vi "ros data.vi"() -> ()   [LabVIEW 2015]
uses:
  Zmienne/szablon odometry_filtered_local.ctl
  TASK ERL/List of robots.ctl
  Zmienne/common msg from UAV-1.vi
  Gobal for ROS.vi
  Zmienne/Lokalizacja GPS/Longitude dron 2.vi
  Zmienne/Lokalizacja GPS/Latitude dron 2.vi
  Zmienne/Lokalizacja GPS/Longitude dron 1.vi
  Zmienne/Lokalizacja GPS/Latitude dron 1.vi
  Zmienne/Lokalizacja GPS/Longitude Sparus.vi
  Zmienne/Lokalizacja GPS/Latitude Sparus.vi
  Zmienne/common msg.vi
  Zmienne/Lokalizacja GPS/azymut.vi
  Zmienne/Lokalizacja GPS/longitude.vi
  Zmienne/Lokalizacja GPS/latitude.vi
  Zmienne/Lokalizacja GPS/longitude Quadron.vi
  Zmienne/Lokalizacja GPS/latitude Quadron.vi
  Zmienne/Lokalizacja GPS/Lokalizacja GPS.lvlib
  KML/KML.lvlib
  TASK ERL/task erl.lvlib
  <vilib>/Intelligent Energy/WebSockets API/WebSockets/WebSockets.lvlib
  ROS.lvlib
  Pomocnicze/Pomocnicze.lvlib
  Matematyczne/Matematyczne.lvlib
  Zmienne/Zmienne.lvlib
panel:
  out "msg.heading 2":dbl
  out "msg.heading":dbl
  in  "AUV-Sparus":path=path "C:/Users/User/Desktop/ERL 2017/TBM1/Surowe dane/Vehicle navigation/AUV-Sparus.txt"
  in  "Common messages":path=path "C:/Users/User/Desktop/ERL 2017/TBM1/Surowe dane/Subtask registered event.txt"
  in  "Tab Control":T1(tab)
  out "raw frame 5":string
  in  "STOP ROS READ 3":bool
  out "Messages read":T2
  out "error out 5":errorcluster
  in  "Topic string 3":string="{ \"op\": \"subscribe\", \"topic\" : \"/common\" }"
  in  "address 2":string="192.168.1.106"
  in  "rosbrige port 3":u16=9090
  in  "ROSB READ 3":bool
  in  "ROSB WRITE":bool
  in  "advertise msg 2":string="{\"op\":\"advertise\", \"topic\":\"common\",\"type\":\"common_msgs/Common\"}"
  out "error out 4":errorcluster
  out "raw frame 4":string="{\"op\":\"\",\"topic\":\"\",\"Msg\":{\"Sender_name\":\"Raptor\",\"Receiver_name\":\"UGV1-Raptor\",\"Latitude\":0,\"Longitude\":0,\"Value_number\":1,\"status\":\"UGV1-Raptor\"}}"
  out "sent messages":T2
  in  "STOP ROS WRITE":bool
  out "ROS data read 4":T3
  in  "ROSB READ\nquadron":bool
  in  "Topic string 2":string="{ \"op\": \"subscribe\", \"topic\" : \"/gps_quadron\" }"
  out "error out 3":errorcluster
  in  "STOP ROS READ\nquadron":bool
  out "raw frame 3":string
  in  "ip":string="192.168.1.117"
  in  "rosbrige port quadron":u16=9091
  in  "ROSB READ \ngps raptor":bool
  in  "ip raptor":string="192.168.1.117"
  in  "rosbrige port raptor":u16=9091
  in  "STOP ROS READ\ngps raptor":bool
  in  "Raptor":enum32{"read GPS ", "read Odometria"}(tab)
  out "raw frame 6":string
  out "error out 6":errorcluster
  in  "Topic string 4":string="{ \"op\": \"subscribe\", \"topic\" : \"/fix\" }"
  out "ROS data read 5":T3
  out "szablon odometry/filtered/local 2":T4
  in  "Topic string 6":string="{ \"op\": \"subscribe\", \"topic\" : \"/odometry/filtered/local\" }"
  out "raw frame 10":string
  out "error out 10":errorcluster
  in  "ROSB READ\nodom raptor":bool
  in  "STOP ROS READ\nodom raptor":bool
  in  "Tab Control 2":T5(tab)
  in  "Topic string 5":string="{ \"op\": \"subscribe\", \"topic\" : \"/drone1/gps\" }"
  out "raw frame 7":string
  out "error out 7":errorcluster
  out "ROS data read 8":T6
  out "value":T7
  out "error out 8":errorcluster
  out "String out":string
  in  "Topic string orientacja":string="{ \"op\": \"subscribe\", \"topic\" : \"/drone1/heading\" }"
  out "raw frame 9":string
  out "Messages read 2":T2
  out "error out 12":errorcluster
  in  "Topic string 8":string="{ \"op\": \"subscribe\", \"topic\" : \"/common\" }"
  in  "advertise msg 3":string="{\"op\":\"advertise\", \"topic\":\"common\",\"type\":\"common_msgs/Common\"}"
  out "error out 9":errorcluster
  out "raw frame 11":string="{\"op\":\"\",\"topic\":\"\",\"Msg\":{\"Sender_name\":\"Raptor\",\"Receiver_name\":\"UGV1-Raptor\",\"Latitude\":0,\"Longitude\":0,\"Value_number\":1,\"status\":\"UGV1-Raptor\"}}"
  in  "ip dron 1":string="192.168.1.106"
  in  "rosbrige port dron 1":u16=9090
  in  "drone 1 gps":bool caption="drone 1 GPS\n position read"
  in  "read drone 1\n gps stop":bool
  in  "read drone 1\nheading read":bool
  in  "read drone 1\n heading stop":bool
  in  "read drone 1\n common":bool
  in  "read drone 1\ncommon stop":bool
  in  "ROSB WRITE \nwrite drone 1 \ncommon":bool
  in  "STOP ROS WRITE \ndron 1 common":bool
  in  "Tab Control 3":T8(tab)
  in  "Topic string 7":string="{ \"op\": \"subscribe\", \"topic\" : \"/drone2/gps\" }"
  out "raw frame 8":string
  out "error out 11":errorcluster
  out "ROS data read 7":T6
  in  "Topic string orientacja 2":string="{ \"op\": \"subscribe\", \"topic\" : \"/drone2/heading\" }"
  out "String out 3":string
  out "error out 13":errorcluster
  out "value 3":T7
  in  "ip dron 2":string="192.168.1.106"
  in  "rosbrige port  dron 2":u16=9090
  in  "ROSB READ \ngps dron 2":bool
  in  "STOP ROS READ \ngps dron 2":bool
  in  "ROSB READ \nheading dron 2":bool
  in  "STOP ROS READ\nheading dron 2":bool
  in  "UAV-2":path=path "C:/Users/User/Desktop/ERL 2017/TBM1/Surowe dane/Vehicle navigation/UAV-2.txt"
  in  "UAV-1":path=path "C:/Users/User/Desktop/ERL 2017/TBM1/Surowe dane/Vehicle navigation/UAV-1.txt"
  in  "UGV2-Quadron":path=path "C:/Users/User/Desktop/ERL 2017/TBM1/Surowe dane/Vehicle navigation/UGV2-Quadron.txt"
  in  "UGV1-Raptor":path=path "C:/Users/User/Desktop/ERL 2017/TBM1/Surowe dane/Vehicle navigation/UGV1-Raptor.txt"
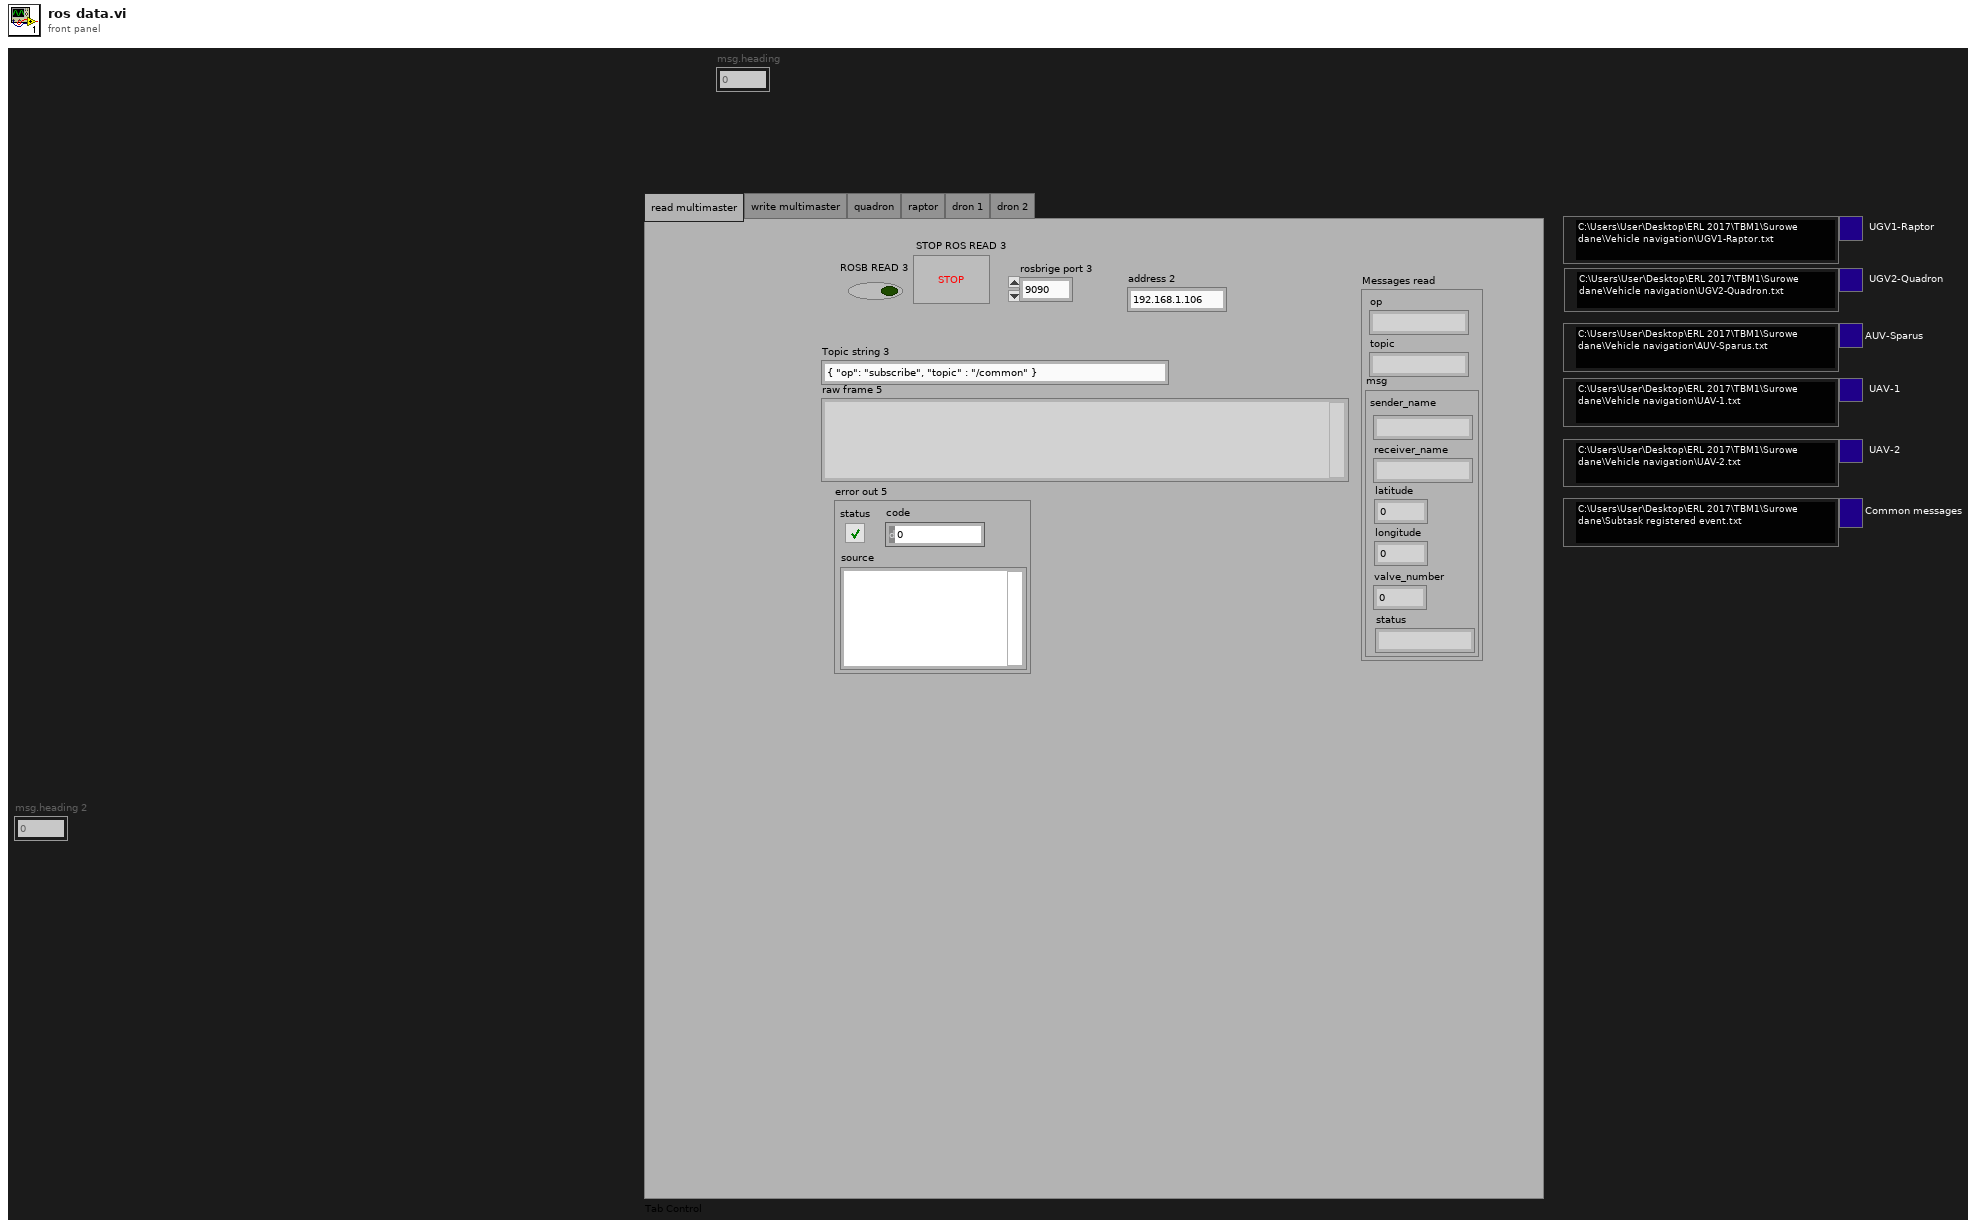
[diagram p1: front panel]
types:
  T1 = enum32{"read multimaster", "write multimaster", "quadron", "raptor", "dron 1", "dron 2"}
  T2 = cluster{"op":string, "topic":string, "msg":cluster{"sender_name":string, "receiver_name":string, "latitude":dbl, "longitude":dbl, "valve_number":i32, "status":string}}
  T3 = cluster{"topic":string, "msg":cluster{"header":cluster{"seq":u32, "stamp":cluster{"secs":u32, "nsecs":i32}, "frame_id":string}, "status":cluster{"status":u32, "service":i32}, "position_covariance":dbl[], "latitude":dbl, "longitude":dbl, "altitude":i32, "position_covariance_type":dbl}, "op":string}
  T4 = typedef "Biblioteka moduł map v3.lvlib/Zmienne.lvlib/szablon odometry_filtered_local.ctl" = cluster{"topic":string, "msg":cluster{"header":cluster{"seq":u32, "stamp":cluster{"secs":u32, "nsecs":i32}, "frame_id":string}, "child_frame_id":string, "pose":cluster{"pose":cluster{"position":cluster{"y":dbl, "z":dbl, "x":dbl}, "orientation":cluster{"y":dbl, "z":dbl, "x":dbl, "w":dbl}}, "covariance":dbl[]}, "twist":cluster{"twist":cluster{"linear":cluster{"y":dbl, "z":dbl, "x":dbl}, "angular":cluster{"y":dbl, "z":dbl, "x":dbl}}, "covariance":dbl[]}}, "op":string}
  T5 = enum32{"read Global position gps", "read heading", "read common", "write common"}
  T6 = cluster{"topic":string, "op":string, "msg":cluster{"header":cluster{"seq":u32, "stamp":cluster{"secs":u32, "nsecs":i32}, "frame_id":string}, "status":cluster{"status":u32, "service":i32}, "position_covariance":dbl[], "latitude":dbl, "longitude":dbl, "altitude":dbl, "position_covariance_type":dbl}}
  T7 = cluster{"topic":string, "op":string, "msg":cluster{"heading":dbl}}
  T8 = enum32{" read Global position gps data", "read heading"}
  T9 = cluster{"topic":string, "msg":cluster{"header":cluster{"seq":u32, "stamp":cluster{"secs":u32, "nsecs":i32}, "frame_id":string}, "child_frame_id":string, "pose":cluster{"pose":cluster{"position":cluster{"y":dbl, "z":dbl, "x":dbl}, "orientation":cluster{"y":dbl, "z":dbl, "x":dbl, "w":dbl}}, "covariance":dbl[]}, "twist":cluster{"twist":cluster{"linear":cluster{"y":dbl, "z":dbl, "x":dbl}, "angular":cluster{"y":dbl, "z":dbl, "x":dbl}}, "covariance":dbl[]}}, "op":string}
  T10 = typedef "Biblioteka moduł map v3.lvlib/task erl.lvlib/List of robots.ctl" = string
  T11 = cluster{"topic":string, "msg":cluster{"header":cluster{"seq":u32, "stamp":cluster{"secs":u32, "nsecs":i32}, "frame_id":string}, "status":cluster{"status":u32, "service":i32}, "position_covariance":dbl[], "latitude":dbl, "longitude":dbl, "altitude":dbl, "position_covariance_type":dbl}, "op":string}
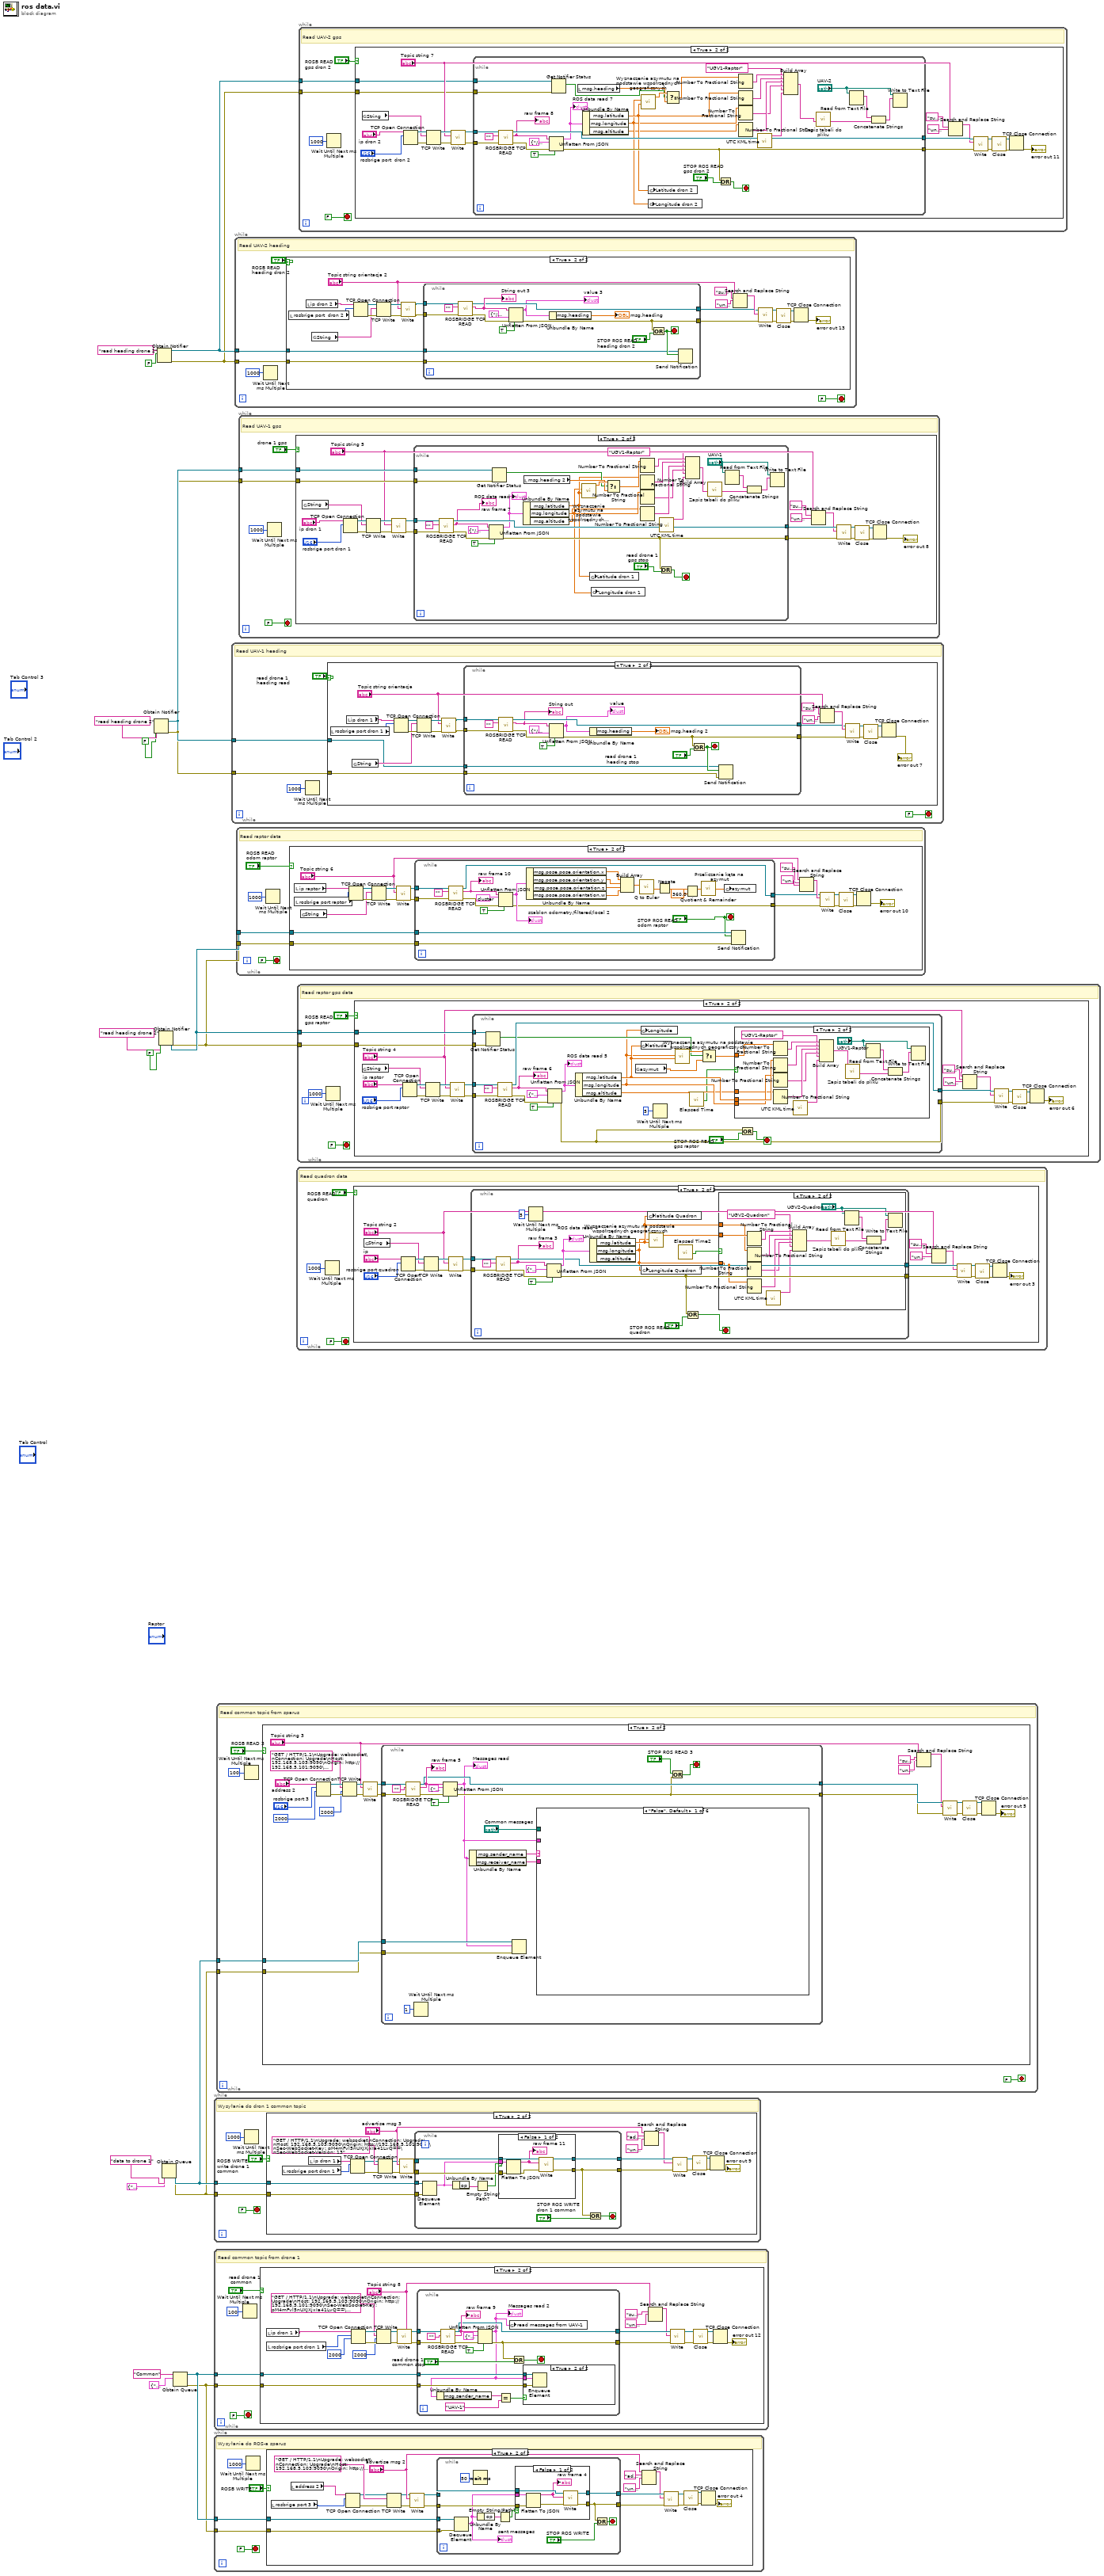
[diagram p0: block diagram]
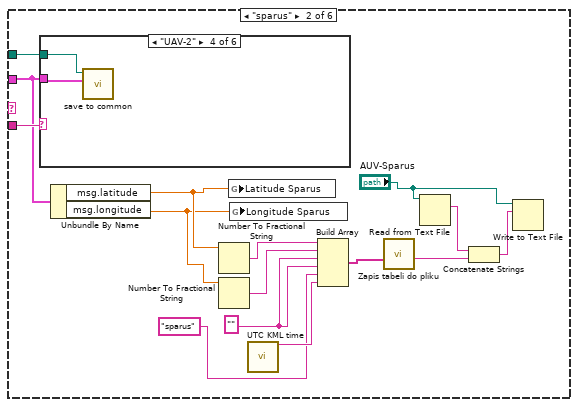
[diagram p13: hidden frame]
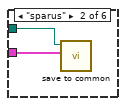
[diagram p15: hidden frame]
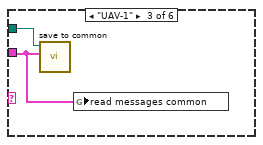
[diagram p16: hidden frame]
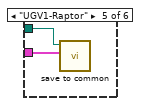
[diagram p17: hidden frame]
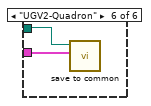
[diagram p18: hidden frame]
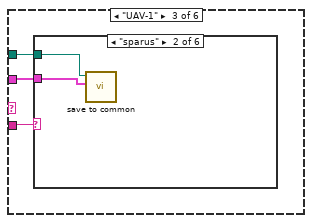
[diagram p19: hidden frame]
diagram:
  n1 = Obtain Notifier(name (unnamed)="read heading drone 2", notification data type=FALSE ("ROSB READ 9")) -> (notifier out=w10:refnum<notifier>, error out=w9:errorcluster)  [unwired: 2 in, 1 out]
  n2 = Obtain Notifier(name (unnamed)="read heading drone 2", notification data type=FALSE ("ROSB READ 9")) -> (notifier out=w16:refnum<notifier>, error out=w15:errorcluster)  [unwired: 2 in, 1 out]
  n3 = Obtain Notifier(name (unnamed)="read heading drone 2", notification data type=FALSE ("ROSB READ 9")) -> (notifier out=w2:refnum<notifier>, error out=w1:errorcluster)  [unwired: 2 in, 1 out]
  n4 = Obtain Queue(name (unnamed)="data to drone 1", element data type=T2 {"op"="", "topic"="", "msg"={"sender_name"="", "receiver_name"="", "latitude"=0.0, "longitude"=0.0, "valve_number"=0, "status"=""}} ("Messages read 3")) -> (queue out=w6:refnum<queue>, error out=w5:errorcluster)  [unwired: 3 in, 1 out]
  n5 = Obtain Queue(name (unnamed)="Common", element data type=T2 {"op"="publish", "topic"="common", "msg"={"sender_name"="", "receiver_name"="", "latitude"=0.0, "longitude"=0.0, "valve_number"=0, "status"=""}} ("Messages read 2")) -> (queue out=w18:refnum<queue>, error out=w17:errorcluster)  [unwired: 3 in, 1 out]
  n6 = while {
    tunnel: w6 -> [w23]
    tunnel: w5 -> [w21]
    stop <- FALSE stop-if-true
    # "Wysyłanie do dron 1 common topic"
    n7 = Wait Until Next ms Multiple(millisecond multiple=u32 1000 ("milliseconds to wait")) -> ()  [unwired: 1 out]
    n8 = case shown="True" "ROSB WRITE \nwrite drone 1 \ncommon" {
      tunnel: w23 -> [_ w29]
      tunnel: w21 -> [_ w28]
      frame False {
      }
      frame True {
        n9 = local read "rosbrige port dron 1"() -> (w26:u16)
        n10 = local read "ip dron 1"() -> (w27:string)
        n11 = TCP Open Connection(address=w27, remote port or service name=w26) -> (connection ID=w33:refnum<k5>, error out=w32:errorcluster)  [unwired: 3 in]
        n12 = TCP Write(connection ID=w33, data in="GET / HTTP/1.1\nUpgrade: websocket\nConnection: Upgrade\nHost: 192.168.5.103:9090\nOrigin: http://192.168.5.101:9090\nSec-WebSocket-Key: pM4mFvl5nUXJXjxIa41LvQ==\nSec-WebSocket-Version: 13", error in (no error)=w32) -> (connection ID out=w31:refnum<k5>, error out=w30:errorcluster)  [unwired: 1 in, 1 out]
        n13 = call <vilib>:"Write.vi"("error in (no error)"=w30, "Data"="advertise msg 3", "WebSocket Connection in"=w31) -> ("error out"=w46:errorcluster, "WebSocket Connection out"=w47:refnum<k5>)  [unwired: 7 in]
        n14 = while {
          tunnel: [w56] -> w39
          tunnel: [w53] -> w38
          tunnel: w47 -> [w57]
          tunnel: w46 -> [w58]
          tunnel: w29 -> [w50]
          tunnel: w28 -> [w49]
          stop <- w51 stop-if-true
          n15 = Dequeue Element(queue=w50, error in (no error)=w49) -> (element=w48:T2)  [unwired: 1 in, 3 out]
          n16 = Unbundle By Name(w48) -> ("op"=w54:string)
          n17 = Empty String/Path?(string/path=w54) -> (empty?=w55:bool)
          n18 = case shown="False" w55 {
            tunnel: w58 -> [w65 w66]
            tunnel: w57 -> [w64 w67]
            tunnel: [w63 w67] -> w56
            tunnel: [w60 w66] -> w53
            tunnel: w48 -> [w59 _]
            frame False {
              n19 = Flatten To JSON(anything=w59, error in (no error)=w65) -> (JSON string=w61:string, 11:w62:errorcluster)  [unwired: 1 in]
              "raw frame 11" <- w61
              n20 = call <vilib>:"Write.vi"("error in (no error)"=w62, "Data"=w61, "WebSocket Connection in"=w64) -> ("error out"=w60:errorcluster, "WebSocket Connection out"=w63:refnum<k5>)  [unwired: 7 in]
            }
            frame True {
            }
          }
          n21 = Or(x=w53, y="STOP ROS WRITE \ndron 1 common") -> (x .or. y?=w51:bool)
        }
        n22 = Search and Replace String(input string="advertise msg 3", search string="advertise", replace string="unadvertise" ("search string")) -> (result string=w34:string)  [unwired: 5 in, 3 out]
        n23 = call <vilib>:"Write.vi"("error in (no error)"=w38, "Data"=w34, "WebSocket Connection in"=w39) -> ("error out"=w40:errorcluster, "WebSocket Connection out"=w41:refnum<k5>)  [unwired: 7 in]
        n24 = call <vilib>:"Close.vi"("error in (no error)"=w40, "WebSocket Connection in"=w41) -> ("error out"=w44:errorcluster, "WebSocket Connection in"=w43:refnum<k5>)  [unwired: 8 in]
        n25 = TCP Close Connection(connection ID=w43, error in (no error)=w44) -> (error out=→"error out 9":errorcluster)  [unwired: 1 in, 1 out]
      }
    }
  }
  n26 = while {
    tunnel: w18 -> [w69]
    tunnel: w17 -> [w68]
    stop <- FALSE stop-if-true
    # "Read common topic from drone 1"
    n27 = Wait Until Next ms Multiple(millisecond multiple=u32 100 ("milliseconds to wait")) -> ()  [unwired: 1 out]
    n28 = case shown="True" "read drone 1\n common" {
      tunnel: w69 -> [_ w76]
      tunnel: w68 -> [_ w75]
      frame False {
      }
      frame True {
        n29 = local read "ip dron 1"() -> (w74:string)
        n30 = local read "rosbrige port dron 1"() -> (w73:u16)
        n31 = TCP Open Connection(address=w74, remote port or service name=w73, timeout ms (60000)=2000) -> (connection ID=w96:refnum<k5>, error out=w95:errorcluster)  [unwired: 2 in]
        n32 = TCP Write(connection ID=w96, data in="GET / HTTP/1.1\nUpgrade: websocket\nConnection: Upgrade\nHost: 192.168.5.103:9090\nOrigin: http://192.168.5.101:9090\nSec-WebSocket-Key: pM4mFvl5nUXJXjxIa41LvQ==\nSec-WebSocket-Version: 13" ("String"), error in (no error)=w95, 9:2000 ("timeout ms (25000)")) -> (connection ID out=w92:refnum<k5>, error out=w91:errorcluster)  [unwired: 1 out]
        n33 = call <vilib>:"Write.vi"("error in (no error)"=w91, "Data"="Topic string 8", "WebSocket Connection in"=w92) -> ("error out"=w89:errorcluster, "WebSocket Connection out"=w90:refnum<k5>)  [unwired: 7 in]
        n34 = while {
          tunnel: [w108] -> w85
          tunnel: [w105] -> w84
          tunnel: w90 -> [w110]
          tunnel: w89 -> [w109]
          tunnel: w76 -> [w102]
          tunnel: w75 -> [w101]
          stop <- w103 stop-if-true
          n35 = call "ROSBRIDGE TCP READ.vi"("error in (no error)"=w109, "String in"="", "TCP Network Connection in"=w110) -> ("error out"=w107:errorcluster, "String out"=w111:string, "TCP Network Connection out"=w108:refnum<k5>)  [unwired: 6 in]
          "raw frame 9" <- w111
          n36 = Unflatten From JSON(JSON string=w111, type and defaults=T2 {"op"="", "topic"="", "msg"={"sender_name"="", "receiver_name"="", "latitude"=0.0, "longitude"=0.0, "valve_number"=0, "status"=""}} ("Messages read 3"), default null elements? (F)=TRUE, error in (no error)=w107) -> (value=w100:T2, error out=w105:errorcluster)  [unwired: 3 in]
          "Messages read 2" <- w100
          n37 = Unbundle By Name(w100) -> ("msg.sender_name"=w99:string)
          n38 = Equal?(x=w99, y="UAV-1") -> (x = y?=w97:bool)
          n39 = global write "common msg from UAV-1.vi" "read messages from UAV-1"(w100) -> ()
          n40 = Or(x=w105, y="read drone 1\ncommon stop") -> (x .or. y?=w103:bool)
          n41 = case shown="True" w97 {
            tunnel: w102 -> [_ w116]
            tunnel: w101 -> [_ w115]
            tunnel: w100 -> [_ w114]
            frame False {
            }
            frame True {
              n42 = Enqueue Element(queue=w116, element=w114, error in (no error)=w115) -> ()  [unwired: 1 in, 3 out]
            }
          }
        }
        n43 = Search and Replace String(input string="Topic string 8", search string="subscribe", replace string="unsubscribe" ("search string")) -> (result string=w83:string)  [unwired: 5 in, 3 out]
        n44 = call <vilib>:"Write.vi"("error in (no error)"=w84, "Data"=w83, "WebSocket Connection in"=w85) -> ("error out"=w86:errorcluster, "WebSocket Connection out"=w87:refnum<k5>)  [unwired: 7 in]
        n45 = call <vilib>:"Close.vi"("error in (no error)"=w86, "WebSocket Connection in"=w87) -> ("error out"=w93:errorcluster, "WebSocket Connection in"=w94:refnum<k5>)  [unwired: 8 in]
        n46 = TCP Close Connection(connection ID=w94, error in (no error)=w93) -> (error out=→"error out 12":errorcluster)  [unwired: 1 in, 1 out]
      }
    }
  }
  n47 = while {
    tunnel: w18 -> [w119]
    tunnel: w17 -> [w117]
    stop <- FALSE stop-if-true
    # "Wysyłanie do ROS-a sparus"
    n48 = Wait Until Next ms Multiple(millisecond multiple=u32 1000 ("milliseconds to wait")) -> ()  [unwired: 1 out]
    n49 = case shown="True" "ROSB WRITE" {
      tunnel: w119 -> [_ w125]
      tunnel: w117 -> [_ w124]
      frame False {
      }
      frame True {
        n50 = local read "rosbrige port 3"() -> (w122:u16)
        n51 = local read "address 2"() -> (w123:string)
        n52 = TCP Open Connection(address=w123, remote port or service name=w122) -> (connection ID=w129:refnum<k5>, error out=w128:errorcluster)  [unwired: 3 in]
        n53 = TCP Write(connection ID=w129, data in="GET / HTTP/1.1\nUpgrade: websocket\nConnection: Upgrade\nHost: 192.168.5.103:9090\nOrigin: http://192.168.5.101:9090\nSec-WebSocket-Key: pM4mFvl5nUXJXjxIa41LvQ==\nSec-WebSocket-Version: 13", error in (no error)=w128) -> (connection ID out=w127:refnum<k5>, error out=w126:errorcluster)  [unwired: 1 in, 1 out]
        n54 = call <vilib>:"Write.vi"("error in (no error)"=w126, "Data"="advertise msg 2", "WebSocket Connection in"=w127) -> ("error out"=w142:errorcluster, "WebSocket Connection out"=w143:refnum<k5>)  [unwired: 7 in]
        n55 = while {
          tunnel: [w153] -> w135
          tunnel: [w146] -> w134
          tunnel: w143 -> [w154]
          tunnel: w142 -> [w155]
          tunnel: w125 -> [w151]
          tunnel: w124 -> [w150]
          stop <- w144 stop-if-true
          n56 = Dequeue Element(queue=w151, error in (no error)=w150) -> (element=w148:T2)  [unwired: 1 in, 3 out]
          "sent messages" <- w148
          n57 = Wait (ms)(milliseconds to wait=u32 50) -> ()  [unwired: 1 out]
          n58 = Unbundle By Name(w148) -> ("op"=w147:string)
          n59 = Empty String/Path?(string/path=w147) -> (empty?=w149:bool)
          n60 = case shown="False" w149 {
            tunnel: w155 -> [w162 w163]
            tunnel: w154 -> [w161 w164]
            tunnel: [w160 w164] -> w153
            tunnel: [w157 w163] -> w146
            tunnel: w148 -> [w156 _]
            frame False {
              n61 = Flatten To JSON(anything=w156, error in (no error)=w162) -> (JSON string=w158:string, 11:w159:errorcluster)  [unwired: 1 in]
              "raw frame 4" <- w158
              n62 = call <vilib>:"Write.vi"("error in (no error)"=w159, "Data"=w158, "WebSocket Connection in"=w161) -> ("error out"=w157:errorcluster, "WebSocket Connection out"=w160:refnum<k5>)  [unwired: 7 in]
            }
            frame True {
            }
          }
          n63 = Or(x=w146, y="STOP ROS WRITE") -> (x .or. y?=w144:bool)
        }
        n64 = Search and Replace String(input string="advertise msg 2", search string="advertise", replace string="unadvertise" ("search string")) -> (result string=w130:string)  [unwired: 5 in, 3 out]
        n65 = call <vilib>:"Write.vi"("error in (no error)"=w134, "Data"=w130, "WebSocket Connection in"=w135) -> ("error out"=w136:errorcluster, "WebSocket Connection out"=w137:refnum<k5>)  [unwired: 7 in]
        n66 = call <vilib>:"Close.vi"("error in (no error)"=w136, "WebSocket Connection in"=w137) -> ("error out"=w140:errorcluster, "WebSocket Connection in"=w139:refnum<k5>)  [unwired: 8 in]
        n67 = TCP Close Connection(connection ID=w139, error in (no error)=w140) -> (error out=→"error out 4":errorcluster)  [unwired: 1 in, 1 out]
      }
    }
  }
  n68 = while {
    tunnel: w6 -> [w166]
    tunnel: w5 -> [w165]
    stop <- FALSE stop-if-true
    # "Read common topic from sparus"
    n69 = Wait Until Next ms Multiple(millisecond multiple=u32 100 ("milliseconds to wait")) -> ()  [unwired: 1 out]
    n70 = case shown="True" "ROSB READ 3" {
      tunnel: w166 -> [_ w171]
      tunnel: w165 -> [_ w170]
      frame False {
      }
      frame True {
        n71 = TCP Open Connection(address="address 2", remote port or service name="rosbrige port 3", timeout ms (60000)=2000) -> (connection ID=w193:refnum<k5>, error out=w192:errorcluster)  [unwired: 2 in]
        n72 = TCP Write(connection ID=w193, data in="GET / HTTP/1.1\nUpgrade: websocket\nConnection: Upgrade\nHost: 192.168.5.103:9090\nOrigin: http://192.168.5.101:9090\nSec-WebSocket-Key: pM4mFvl5nUXJXjxIa41LvQ==\nSec-WebSocket-Version: 13" ("String"), error in (no error)=w192, 9:2000 ("timeout ms (25000)")) -> (connection ID out=w189:refnum<k5>, error out=w188:errorcluster)  [unwired: 1 out]
        n73 = call <vilib>:"Write.vi"("error in (no error)"=w188, "Data"="Topic string 3", "WebSocket Connection in"=w189) -> ("error out"=w186:errorcluster, "WebSocket Connection out"=w187:refnum<k5>)  [unwired: 7 in]
        n74 = while {
          tunnel: [w206] -> w182
          tunnel: [w199] -> w181
          tunnel: w187 -> [w208]
          tunnel: w186 -> [w207]
          tunnel: w171 -> [w197]
          tunnel: w170 -> [w196]
          stop <- w198 stop-if-true
          n75 = call "ROSBRIDGE TCP READ.vi"("error in (no error)"=w207, "String in"="", "TCP Network Connection in"=w208) -> ("error out"=w205:errorcluster, "String out"=w209:string, "TCP Network Connection out"=w206:refnum<k5>)  [unwired: 6 in]
          "raw frame 5" <- w209
          n76 = Wait Until Next ms Multiple(millisecond multiple=u32 1) -> ()  [unwired: 1 out]
          n77 = Unflatten From JSON(JSON string=w209, type and defaults=T2 {"op"="", "topic"="", "msg"={"sender_name"="", "receiver_name"="", "latitude"=0.0, "longitude"=0.0, "valve_number"=0, "status"=""}} ("Messages read 3"), default null elements? (F)=TRUE, error in (no error)=w205) -> (value=w195:T2, error out=w199:errorcluster)  [unwired: 3 in]
          "Messages read" <- w195
          n78 = Unbundle By Name(w195) -> ("msg.sender_name"=w203:string, "msg.receiver_name"=w194:string)
          n79 = Enqueue Element(queue=w197, element=w195, error in (no error)=w196) -> ()  [unwired: 1 in, 3 out]
          n80 = case shown="\"False\", Default" w203 {
            selector: w203 -> [_ _ _ _ _ w279]
            tunnel: "Common messages" -> [_ w226 w239 w250 w265 w278]
            tunnel: w195 -> [_ w221 w238 w251 w264 w277]
            tunnel: w194 -> [_ w225 w237 w252 w263 w276]
            frame "False", Default {
            }
            frame "sparus" {
              w217 = "" ("element")
              n81 = case shown="\"UAV-2\"" w225 {
                tunnel: w226 -> [_ w228 w230 w231 w233 w236]
                tunnel: w221 -> [_ w227 w229 w232 w234 w235]
                frame "False", Default {
                }
                frame "sparus" {
                  n82 = call "save to common.vi"("Messages read 3"=w227, "Common messages"=w228) -> ()  [unwired: 9 in]
                }
                frame "UAV-1" {
                  n83 = call "save to common.vi"("Messages read 3"=w229, "Common messages"=w230) -> ()  [unwired: 9 in]
                  n84 = global write "common msg.vi" "read messages common"(w229) -> ()
                }
                frame "UAV-2" {
                  n85 = call "save to common.vi"("Messages read 3"=w232, "Common messages"=w231) -> ()  [unwired: 9 in]
                }
                frame "UGV1-Raptor" {
                  n86 = call "save to common.vi"("Messages read 3"=w234, "Common messages"=w233) -> ()  [unwired: 9 in]
                }
                frame "UGV2-Quadron" {
                  n87 = call "save to common.vi"("Messages read 3"=w235, "Common messages"=w236) -> ()  [unwired: 9 in]
                }
              }
              n88 = Unbundle By Name(w221) -> ("msg.latitude"=w216:dbl, "msg.longitude"=w215:dbl)
              n89 = Number To Fractional String(number=w216) -> (F-format string=w220:string)  [unwired: 3 in]
              n90 = Number To Fractional String(number=w215) -> (F-format string=w219:string)  [unwired: 3 in]
              n91 = global write "Latitude Sparus.vi" "Latitude Sparus"(w216) -> ()
              n92 = global write "Longitude Sparus.vi" "Longitude Sparus"(w215) -> ()
              n93 = call "UTC KML time.vi"() -> ("String"=w214:string)  [unwired: 19 in]
              n94 = Build Array(w220, w219, w217, w217, "sparus" ("element"), w214) -> (w218:string[])
              n95 = call "Zapis tabeli do pliku.vi"("1d array in"=w218) -> ("for 1d array out"=w222:string)  [unwired: 7 in, 1 out]
              n96 = Read from Text File(file (use dialog)="AUV-Sparus") -> (text=w224:string)  [unwired: 3 in, 3 out]
              n97 = Concatenate Strings(w224, w222) -> (w223:string)
              n98 = Write to Text File(file (use dialog)="AUV-Sparus", text=w223) -> ()  [unwired: 2 in, 3 out]
            }
            frame "UAV-1" {
              n99 = case shown="\"sparus\"" w237 {
                tunnel: w239 -> [_ w241 w243 w244 w246 w249]
                tunnel: w238 -> [_ w240 w242 w245 w247 w248]
                frame "False", Default {
                }
                frame "sparus" {
                  n100 = call "save to common.vi"("Messages read 3"=w240, "Common messages"=w241) -> ()  [unwired: 9 in]
                }
                frame "UAV-1" {
                  n101 = call "save to common.vi"("Messages read 3"=w242, "Common messages"=w243) -> ()  [unwired: 9 in]
                  n102 = global write "common msg from UAV-1.vi" "read messages from UAV-1"(w242) -> ()
                }
                frame "UAV-2" {
                  n103 = call "save to common.vi"("Messages read 3"=w245, "Common messages"=w244) -> ()  [unwired: 9 in]
                }
                frame "UGV1-Raptor" {
                  n104 = call "save to common.vi"("Messages read 3"=w247, "Common messages"=w246) -> ()  [unwired: 9 in]
                }
                frame "UGV2-Quadron" {
                  n105 = call "save to common.vi"("Messages read 3"=w248, "Common messages"=w249) -> ()  [unwired: 9 in]
                }
              }
            }
            frame "UAV-2" {
              n106 = case shown="\"False\", Default" w252 {
                tunnel: w250 -> [_ w254 w255 w257 w259 w262]
                tunnel: w251 -> [_ w253 w256 w258 w260 w261]
                frame "False", Default {
                }
                frame "sparus" {
                  n107 = call "save to common.vi"("Messages read 3"=w253, "Common messages"=w254) -> ()  [unwired: 9 in]
                }
                frame "UAV-1" {
                  n108 = call "save to common.vi"("Messages read 3"=w256, "Common messages"=w255) -> ()  [unwired: 9 in]
                }
                frame "UAV-2" {
                  n109 = call "save to common.vi"("Messages read 3"=w258, "Common messages"=w257) -> ()  [unwired: 9 in]
                }
                frame "UGV1-Raptor" {
                  n110 = call "save to common.vi"("Messages read 3"=w260, "Common messages"=w259) -> ()  [unwired: 9 in]
                }
                frame "UGV2-Quadron" {
                  n111 = call "save to common.vi"("Messages read 3"=w261, "Common messages"=w262) -> ()  [unwired: 9 in]
                }
              }
            }
            frame "UGV1-Raptor" {
              n112 = case shown="\"False\", Default" w263 {
                tunnel: w265 -> [_ w267 w268 w270 w272 w275]
                tunnel: w264 -> [_ w266 w269 w271 w273 w274]
                frame "False", Default {
                }
                frame "sparus" {
                  n113 = call "save to common.vi"("Messages read 3"=w266, "Common messages"=w267) -> ()  [unwired: 9 in]
                }
                frame "UAV-1" {
                  n114 = call "save to common.vi"("Messages read 3"=w269, "Common messages"=w268) -> ()  [unwired: 9 in]
                }
                frame "UAV-2" {
                  n115 = call "save to common.vi"("Messages read 3"=w271, "Common messages"=w270) -> ()  [unwired: 9 in]
                }
                frame "UGV1-Raptor" {
                  n116 = call "save to common.vi"("Messages read 3"=w273, "Common messages"=w272) -> ()  [unwired: 9 in]
                }
                frame "UGV2-Quadron" {
                  n117 = call "save to common.vi"("Messages read 3"=w274, "Common messages"=w275) -> ()  [unwired: 9 in]
                }
              }
            }
            frame "UGV2-Quadron" {
              n118 = case shown="\"False\", Default" w276 {
                tunnel: w279 -> [_ _ _ _ _ _]
                tunnel: w278 -> [_ w281 w282 w284 w286 w289]
                tunnel: w277 -> [_ w280 w283 w285 w287 w288]
                frame "False", Default {
                }
                frame "sparus" {
                  n119 = call "save to common.vi"("Messages read 3"=w280, "Common messages"=w281) -> ()  [unwired: 9 in]
                }
                frame "UAV-1" {
                  n120 = call "save to common.vi"("Messages read 3"=w283, "Common messages"=w282) -> ()  [unwired: 9 in]
                }
                frame "UAV-2" {
                  n121 = call "save to common.vi"("Messages read 3"=w285, "Common messages"=w284) -> ()  [unwired: 9 in]
                }
                frame "UGV1-Raptor" {
                  n122 = call "save to common.vi"("Messages read 3"=w287, "Common messages"=w286) -> ()  [unwired: 9 in]
                }
                frame "UGV2-Quadron" {
                  n123 = call "save to common.vi"("Messages read 3"=w288, "Common messages"=w289) -> ()  [unwired: 9 in]
                }
              }
            }
          }
          n124 = Or(x="STOP ROS READ 3", y=w199) -> (x .or. y?=w198:bool)
        }
        n125 = Search and Replace String(input string="Topic string 3", search string="subscribe", replace string="unsubscribe" ("search string")) -> (result string=w180:string)  [unwired: 5 in, 3 out]
        n126 = call <vilib>:"Write.vi"("error in (no error)"=w181, "Data"=w180, "WebSocket Connection in"=w182) -> ("error out"=w183:errorcluster, "WebSocket Connection out"=w184:refnum<k5>)  [unwired: 7 in]
        n127 = call <vilib>:"Close.vi"("error in (no error)"=w183, "WebSocket Connection in"=w184) -> ("error out"=w190:errorcluster, "WebSocket Connection in"=w191:refnum<k5>)  [unwired: 8 in]
        n128 = TCP Close Connection(connection ID=w191, error in (no error)=w190) -> (error out=→"error out 5":errorcluster)  [unwired: 1 in, 1 out]
      }
    }
  }
  n129 = while {
    tunnel: w10 -> [w291]
    tunnel: w9 -> [w290]
    stop <- FALSE stop-if-true
    # "Read UAV-1 heading"
    n130 = Wait Until Next ms Multiple(millisecond multiple=u32 1000 ("milliseconds to wait")) -> ()  [unwired: 1 out]
    n131 = case shown="True" "read drone 1\nheading read" {
      tunnel: w291 -> [_ w298]
      tunnel: w290 -> [_ w297]
      frame False {
      }
      frame True {
        n132 = local read "rosbrige port dron 1"() -> (w299:u16)
        n133 = local read "ip dron 1"() -> (w300:string)
        n134 = global read "Gobal for ROS.vi" "String"() -> (w312:string)
        n135 = TCP Open Connection(address=w300, remote port or service name=w299) -> (connection ID=w313:refnum<k5>, error out=w314:errorcluster)  [unwired: 3 in]
        n136 = TCP Write(connection ID=w313, data in=w312, error in (no error)=w314) -> (connection ID out=w315:refnum<k5>, error out=w316:errorcluster)  [unwired: 1 in, 1 out]
        n137 = call <vilib>:"Write.vi"("error in (no error)"=w316, "Data"="Topic string orientacja", "WebSocket Connection in"=w315) -> ("error out"=w303:errorcluster, "WebSocket Connection out"=w304:refnum<k5>)  [unwired: 7 in]
        n138 = while {
          tunnel: w304 -> [w328]
          tunnel: w303 -> [w327]
          tunnel: [w326] -> w302
          tunnel: [w323] -> w301
          tunnel: w298 -> [w320]
          tunnel: w297 -> [w319]
          stop <- w321 stop-if-true
          n139 = call "ROSBRIDGE TCP READ.vi"("error in (no error)"=w327, "String in"="", "TCP Network Connection in"=w328) -> ("error out"=w330:errorcluster, "String out"=w317:string, "TCP Network Connection out"=w326:refnum<k5>)  [unwired: 6 in]
          "String out" <- w317
          n140 = Unflatten From JSON(JSON string=w317, type and defaults=T7 {"topic"="/mavros/global_position/global", "op"="publish", "msg"={"heading"=47.3977415}} ("ROS data read 7"), default null elements? (F)=TRUE, error in (no error)=w330) -> (value=w318:T7, error out=w323:errorcluster)  [unwired: 3 in]
          "value" <- w318
          n141 = Unbundle By Name(w318) -> ("msg.heading"=→"msg.heading 2":dbl)
          n142 = Or(x=w323, y="read drone 1\n heading stop") -> (x .or. y?=w321:bool)
          n143 = Send Notification(notification=w321, notifier=w320, error in (no error)=w319) -> ()  [unwired: 2 out]
        }
        n144 = Search and Replace String(input string="Topic string orientacja", search string="subscribe", replace string="unsubscribe" ("search string")) -> (result string=w309:string)  [unwired: 5 in, 3 out]
        n145 = call <vilib>:"Write.vi"("error in (no error)"=w301, "Data"=w309, "WebSocket Connection in"=w302) -> ("error out"=w308:errorcluster, "WebSocket Connection out"=w307:refnum<k5>)  [unwired: 7 in]
        n146 = call <vilib>:"Close.vi"("error in (no error)"=w308, "WebSocket Connection in"=w307) -> ("error out"=w306:errorcluster, "WebSocket Connection in"=w305:refnum<k5>)  [unwired: 8 in]
        n147 = TCP Close Connection(connection ID=w305, error in (no error)=w306) -> (error out=→"error out 7":errorcluster)  [unwired: 1 in, 1 out]
      }
    }
  }
  n148 = while {
    tunnel: w16 -> [w333]
    tunnel: w15 -> [w332]
    stop <- FALSE stop-if-true
    # "Read UAV-2 heading"
    n149 = Wait Until Next ms Multiple(millisecond multiple=u32 1000 ("milliseconds to wait")) -> ()  [unwired: 1 out]
    n150 = case shown="True" "ROSB READ \nheading dron 2" {
      tunnel: w333 -> [_ w338]
      tunnel: w332 -> [_ w337]
      frame False {
      }
      frame True {
        n151 = local read "rosbrige port  dron 2"() -> (w339:u16)
        n152 = local read "ip dron 2"() -> (w340:string)
        n153 = global read "Gobal for ROS.vi" "String"() -> (w354:string)
        n154 = TCP Open Connection(address=w340, remote port or service name=w339) -> (connection ID=w355:refnum<k5>, error out=w356:errorcluster)  [unwired: 3 in]
        n155 = TCP Write(connection ID=w355, data in=w354, error in (no error)=w356) -> (connection ID out=w357:refnum<k5>, error out=w358:errorcluster)  [unwired: 1 in, 1 out]
        n156 = call <vilib>:"Write.vi"("error in (no error)"=w358, "Data"="Topic string orientacja 2", "WebSocket Connection in"=w357) -> ("error out"=w344:errorcluster, "WebSocket Connection out"=w345:refnum<k5>)  [unwired: 7 in]
        n157 = while {
          tunnel: w345 -> [w369]
          tunnel: w344 -> [w368]
          tunnel: [w367] -> w343
          tunnel: [w363] -> w342
          tunnel: w338 -> [w360]
          tunnel: w337 -> [w359]
          stop <- w361 stop-if-true
          n158 = call "ROSBRIDGE TCP READ.vi"("error in (no error)"=w368, "String in"="", "TCP Network Connection in"=w369) -> ("error out"=w371:errorcluster, "String out"=w373:string, "TCP Network Connection out"=w367:refnum<k5>)  [unwired: 6 in]
          "String out 3" <- w373
          n159 = Unflatten From JSON(JSON string=w373, type and defaults=T7 {"topic"="/mavros/global_position/global", "op"="publish", "msg"={"heading"=47.3977415}} ("ROS data read 7"), default null elements? (F)=TRUE, error in (no error)=w371) -> (value=w365:T7, error out=w363:errorcluster)  [unwired: 3 in]
          "value 3" <- w365
          n160 = Unbundle By Name(w365) -> ("msg.heading"=→"msg.heading":dbl)
          n161 = Or(x=w363, y="STOP ROS READ\nheading dron 2") -> (x .or. y?=w361:bool)
          n162 = Send Notification(notification=w361, notifier=w360, error in (no error)=w359) -> ()  [unwired: 2 out]
        }
        n163 = Search and Replace String(input string="Topic string orientacja 2", search string="subscribe", replace string="unsubscribe" ("search string")) -> (result string=w351:string)  [unwired: 5 in, 3 out]
        n164 = call <vilib>:"Write.vi"("error in (no error)"=w342, "Data"=w351, "WebSocket Connection in"=w343) -> ("error out"=w350:errorcluster, "WebSocket Connection out"=w349:refnum<k5>)  [unwired: 7 in]
        n165 = call <vilib>:"Close.vi"("error in (no error)"=w350, "WebSocket Connection in"=w349) -> ("error out"=w348:errorcluster, "WebSocket Connection in"=w347:refnum<k5>)  [unwired: 8 in]
        n166 = TCP Close Connection(connection ID=w347, error in (no error)=w348) -> (error out=→"error out 13":errorcluster)  [unwired: 1 in, 1 out]
      }
    }
  }
  n167 = while {
    tunnel: w2 -> [w375]
    tunnel: w1 -> [w374]
    stop <- FALSE stop-if-true
    # "Read raptor data"
    n168 = Wait Until Next ms Multiple(millisecond multiple=u32 1000 ("milliseconds to wait")) -> ()  [unwired: 1 out]
    n169 = case shown="True" "ROSB READ\nodom raptor" {
      tunnel: w375 -> [_ w380]
      tunnel: w374 -> [_ w379]
      frame False {
      }
      frame True {
        n170 = local read "ip raptor"() -> (w383:string)
        n171 = local read "rosbrige port raptor"() -> (w384:u16)
        n172 = global read "Gobal for ROS.vi" "String"() -> (w396:string)
        n173 = TCP Open Connection(address=w383, remote port or service name=w384) -> (connection ID=w397:refnum<k5>, error out=w398:errorcluster)  [unwired: 3 in]
        n174 = TCP Write(connection ID=w397, data in=w396, error in (no error)=w398) -> (connection ID out=w399:refnum<k5>, error out=w400:errorcluster)  [unwired: 1 in, 1 out]
        n175 = call <vilib>:"Write.vi"("error in (no error)"=w400, "Data"="Topic string 6", "WebSocket Connection in"=w399) -> ("error out"=w387:errorcluster, "WebSocket Connection out"=w388:refnum<k5>)  [unwired: 7 in]
        n176 = while {
          tunnel: w388 -> [w420]
          tunnel: w387 -> [w419]
          tunnel: [w408] -> w386
          tunnel: [w418] -> w385
          tunnel: w380 -> [w410]
          tunnel: w379 -> [w409]
          stop <- "STOP ROS READ\nodom raptor" stop-if-true
          n177 = call "ROSBRIDGE TCP READ.vi"("error in (no error)"=w419, "String in"="", "TCP Network Connection in"=w420) -> ("error out"=w422:errorcluster, "String out"=w412:string, "TCP Network Connection out"=w418:refnum<k5>)  [unwired: 6 in]
          "raw frame 10" <- w412
          n178 = Unflatten From JSON(JSON string=w412, type and defaults=T9 {"topic"="", "msg"={"header"={"seq"=0, "stamp"={"secs"=0, "nsecs"=0}, "frame_id"=""}, "child_frame_id"="", "pose"={"pose"={"position"={"y"=0.0, "z"=0.0, "x"=0.0}, "orientation"={"y"=0.0, "z"=0.0, "x"=0.0, "w"=0.0}}, "covariance"=[]}, "twist"={"twist"={"linear"={"y"=0.0, "z"=0.0, "x"=0.0}, "angular"={"y"=0.0, "z"=0.0, "x"=0.0}}, "covariance"=[]}}, "op"=""} ("szablon odometry/filtered/local"), default null elements? (F)=TRUE, error in (no error)=w422) -> (value=w411:T9, error out=w408:errorcluster)  [unwired: 3 in]
          "szablon odometry/filtered/local 2" <- w411
          n179 = Unbundle By Name(w411) -> ("msg.pose.pose.orientation.x"=w404:dbl, "msg.pose.pose.orientation.y"=w403:dbl, "msg.pose.pose.orientation.z"=w402:dbl, "msg.pose.pose.orientation.w"=w401:dbl)
          n180 = Build Array(w404, w403, w402, w401) -> (w405:dbl[])
          n181 = call "Q to Euler.vi"("array"=w405) -> ("Yaw"=w414:dbl)  [unwired: 3 in, 3 out]
          n182 = Negate(x=w414) -> (-x=w415:dbl)
          n183 = Quotient & Remainder(x=w415, y=360.0) -> (x-y*floor(x/y)=w417:dbl)  [unwired: 1 out]
          n184 = call "Przeliczanie kąta na azymut.vi"("Kąt [stoponie]"=w417) -> ("Azymut [stopnie]"=w406:dbl)  [unwired: 4 in]
          n185 = global write "azymut.vi" "azymut"(w406) -> ()
          n186 = Send Notification(notification="STOP ROS READ\nodom raptor", notifier=w410, error in (no error)=w409) -> ()  [unwired: 2 out]
        }
        n187 = Search and Replace String(input string="Topic string 6", search string="subscribe", replace string="unsubscribe" ("search string")) -> (result string=w393:string)  [unwired: 5 in, 3 out]
        n188 = call <vilib>:"Write.vi"("error in (no error)"=w386, "Data"=w393, "WebSocket Connection in"=w385) -> ("error out"=w392:errorcluster, "WebSocket Connection out"=w391:refnum<k5>)  [unwired: 7 in]
        n189 = call <vilib>:"Close.vi"("error in (no error)"=w392, "WebSocket Connection in"=w391) -> ("error out"=w390:errorcluster, "WebSocket Connection in"=w389:refnum<k5>)  [unwired: 8 in]
        n190 = TCP Close Connection(connection ID=w389, error in (no error)=w390) -> (error out=→"error out 10":errorcluster)  [unwired: 1 in, 1 out]
      }
    }
  }
  n191 = while {
    tunnel: w10 -> [w426]
    tunnel: w9 -> [w425]
    stop <- FALSE stop-if-true
    # "Read UAV-1 gps"
    n192 = Wait Until Next ms Multiple(millisecond multiple=u32 1000 ("milliseconds to wait")) -> ()  [unwired: 1 out]
    n193 = case shown="True" "drone 1 gps" {
      tunnel: w426 -> [_ w434]
      tunnel: w425 -> [_ w433]
      frame False {
      }
      frame True {
        n194 = global read "Gobal for ROS.vi" "String"() -> (w435:string)
        n195 = TCP Open Connection(address="ip dron 1", remote port or service name="rosbrige port dron 1") -> (connection ID=w450:refnum<k5>, error out=w449:errorcluster)  [unwired: 3 in]
        n196 = TCP Write(connection ID=w450, data in=w435, error in (no error)=w449) -> (connection ID out=w446:refnum<k5>, error out=w445:errorcluster)  [unwired: 1 in, 1 out]
        n197 = call <vilib>:"Write.vi"("error in (no error)"=w445, "Data"="Topic string 5", "WebSocket Connection in"=w446) -> ("error out"=w443:errorcluster, "WebSocket Connection out"=w444:refnum<k5>)  [unwired: 7 in]
        n198 = while {
          tunnel: [w480] -> w440
          tunnel: [w474] -> w439
          tunnel: w444 -> [w481]
          tunnel: w443 -> [w478]
          tunnel: w434 -> [w471]
          tunnel: w433 -> [w470]
          stop <- w472 stop-if-true
          n199 = call "ROSBRIDGE TCP READ.vi"("error in (no error)"=w478, "String in"="", "TCP Network Connection in"=w481) -> ("error out"=w479:errorcluster, "String out"=w468:string, "TCP Network Connection out"=w480:refnum<k5>)  [unwired: 6 in]
          "raw frame 7" <- w468
          n200 = Unflatten From JSON(JSON string=w468, type and defaults=T6 {"topic"="/drone1/gps", "op"="publish", "msg"={"header"={"seq"=404, "stamp"={"secs"=1505897851, "nsecs"=832105807}, "frame_id"="fcu"}, "status"={"status"=0, "service"=1}, "position_covariance"=[0.0, 0.0, 0.0, 0.0, 0.0, 0.0, 0.0, 0.0, 0.0], "latitude"=47.3977423, "longitude"=8.5455944, "altitude"=0.08040245622396469, "position_covariance_type"=1.0}} ("ROS data read 8"), default null elements? (F)=TRUE, error in (no error)=w479) -> (value=w466:T6, error out=w474:errorcluster)  [unwired: 3 in]
          "ROS data read 8" <- w466
          n201 = Get Notifier Status(notifier=w471, error in (no error)=w470) -> (current notification=w469:bool)  [unwired: 4 out]
          n202 = Unbundle By Name(w466) -> ("msg.latitude"=w454:dbl, "msg.longitude"=w453:dbl, "msg.altitude"=w452:dbl)
          n203 = local read "msg.heading 2"() -> (w475:dbl)
          n204 = call "Wyznaczenie azymutu na podstawie współrzędnych geograficznych.vi"("latitude"=w454, "Longitude"=w453) -> ("Azymut robota\n pocz/nowy 2"=w476:dbl)  [unwired: 9 in]
          n205 = global write "Latitude dron 1.vi" "Latitude dron 1"(w454) -> ()
          n206 = global write "Longitude dron 1.vi" "Longitude dron 1"(w453) -> ()
          n207 = Select(t=w476, s=w469, f=w475) -> (s? t:f=w456:dbl)
          n208 = Number To Fractional String(number=w456) -> (F-format string=w461:string)  [unwired: 3 in]
          n209 = Number To Fractional String(number=w454) -> (F-format string=w460:string)  [unwired: 3 in]
          n210 = Number To Fractional String(number=w453) -> (F-format string=w458:string)  [unwired: 3 in]
          n211 = Number To Fractional String(number=w452) -> (F-format string=w459:string)  [unwired: 3 in]
          n212 = Or(x=w474, y="read drone 1\n gps stop") -> (x .or. y?=w472:bool)
          n213 = call "UTC KML time.vi"() -> ("String"=w457:string)  [unwired: 19 in]
          n214 = Build Array(w461, w460, w459, w458, T10 "UGV1-Raptor" ("List of robots"), w457) -> (w451:T10[])
          n215 = call "Zapis tabeli do pliku.vi"("1d array in"=w451) -> ("for 1d array out"=w465:string)  [unwired: 7 in, 1 out]
          n216 = Read from Text File(file (use dialog)="UAV-1") -> (text=w462:string)  [unwired: 3 in, 3 out]
          n217 = Concatenate Strings(w462, w465) -> (w463:string)
          n218 = Write to Text File(file (use dialog)="UAV-1", text=w463) -> ()  [unwired: 2 in, 3 out]
        }
        n219 = Search and Replace String(input string="Topic string 5", search string="subscribe", replace string="unsubscribe" ("search string")) -> (result string=w438:string)  [unwired: 5 in, 3 out]
        n220 = call <vilib>:"Write.vi"("error in (no error)"=w439, "Data"=w438, "WebSocket Connection in"=w440) -> ("error out"=w441:errorcluster, "WebSocket Connection out"=w442:refnum<k5>)  [unwired: 7 in]
        n221 = call <vilib>:"Close.vi"("error in (no error)"=w441, "WebSocket Connection in"=w442) -> ("error out"=w447:errorcluster, "WebSocket Connection in"=w448:refnum<k5>)  [unwired: 8 in]
        n222 = TCP Close Connection(connection ID=w448, error in (no error)=w447) -> (error out=→"error out 8":errorcluster)  [unwired: 1 in, 1 out]
      }
    }
  }
  n223 = while {
    stop <- FALSE stop-if-true
    # "Read quadron data"
    n224 = Wait Until Next ms Multiple(millisecond multiple=u32 1000 ("milliseconds to wait")) -> ()  [unwired: 1 out]
    n225 = case shown="True" "ROSB READ\nquadron" {
      frame False {
      }
      frame True {
        n226 = global read "Gobal for ROS.vi" "String"() -> (w496:string)
        n227 = TCP Open Connection(address="ip", remote port or service name="rosbrige port quadron") -> (connection ID=w505:refnum<k5>, error out=w504:errorcluster)  [unwired: 3 in]
        n228 = TCP Write(connection ID=w505, data in=w496, error in (no error)=w504) -> (connection ID out=w501:refnum<k5>, error out=w500:errorcluster)  [unwired: 1 in, 1 out]
        n229 = call <vilib>:"Write.vi"("error in (no error)"=w500, "Data"="Topic string 2", "WebSocket Connection in"=w501) -> ("error out"=w498:errorcluster, "WebSocket Connection out"=w499:refnum<k5>)  [unwired: 7 in]
        n230 = while {
          tunnel: [w518] -> w493
          tunnel: [w506] -> w492
          tunnel: w499 -> [w519]
          tunnel: w498 -> [w515]
          stop <- w512 stop-if-true
          n231 = call "ROSBRIDGE TCP READ.vi"("error in (no error)"=w515, "String in"="", "TCP Network Connection in"=w519) -> ("error out"=w516:errorcluster, "String out"=w517:string, "TCP Network Connection out"=w518:refnum<k5>)  [unwired: 6 in]
          "raw frame 3" <- w517
          n232 = Wait Until Next ms Multiple(millisecond multiple=u32 5) -> ()  [unwired: 1 out]
          n233 = Unflatten From JSON(JSON string=w517, type and defaults=T11 {"topic"="", "msg"={"header"={"seq"=0, "stamp"={"secs"=0, "nsecs"=0}, "frame_id"=""}, "status"={"status"=0, "service"=0}, "position_covariance"=[], "latitude"=0.0, "longitude"=0.0, "altitude"=0.0, "position_covariance_type"=0.0}, "op"=""} ("ROS data read 3"), default null elements? (F)=TRUE, error in (no error)=w516) -> (value=w520:T11, error out=w506:errorcluster)  [unwired: 3 in]
          "ROS data read 4" <- w520
          n234 = Unbundle By Name(w520) -> ("msg.latitude"=w510:dbl, "msg.longitude"=w509:dbl)  [unwired: 1 out]
          n235 = global write "longitude Quadron.vi" "Longitude Quadron"(w509) -> ()
          n236 = global write "latitude Quadron.vi" "latitude Quadron"(w510) -> ()
          n237 = call "Wyznaczenie azymutu na podstawie współrzędnych geograficznych.vi"("latitude"=w510, "Longitude"=w509) -> ("Azymut robota\n pocz/nowy 2"=w511:dbl)  [unwired: 9 in]
          n238 = call "Elapsed Time2"() -> ("Time has Elapsed"=w508:bool)  [unwired: 12 in, 7 out]
          n239 = Or(x=w506, y="STOP ROS READ\nquadron") -> (x .or. y?=w512:bool)
          n240 = case shown="True" w508 {
            tunnel: w511 -> [_ w525]
            tunnel: w510 -> [_ w524]
            tunnel: w509 -> [_ w523]
            frame False {
            }
            frame True {
              n241 = Number To Fractional String(number=w525) -> (F-format string=w535:string)  [unwired: 3 in]
              n242 = Number To Fractional String(number=w524) -> (F-format string=w534:string)  [unwired: 3 in]
              n243 = Number To Fractional String(number=w523) -> (F-format string=w532:string)  [unwired: 3 in]
              n244 = Number To Fractional String(number=w523) -> (F-format string=w533:string)  [unwired: 3 in]
              n245 = call "UTC KML time.vi"() -> ("String"=w531:string)  [unwired: 19 in]
              n246 = Build Array(w535, w534, w533, w532, T10 "UGV2-Quadron" ("List of robots"), w531) -> (w536:T10[])
              n247 = call "Zapis tabeli do pliku.vi"("1d array in"=w536) -> ("for 1d array out"=w527:string)  [unwired: 7 in, 1 out]
              n248 = Read from Text File(file (use dialog)="UGV2-Quadron") -> (text=w530:string)  [unwired: 3 in, 3 out]
              n249 = Concatenate Strings(w530, w527) -> (w529:string)
              n250 = Write to Text File(file (use dialog)="UGV2-Quadron", text=w529) -> ()  [unwired: 2 in, 3 out]
            }
          }
        }
        n251 = Search and Replace String(input string="Topic string 2", search string="subscribe", replace string="unsubscribe" ("search string")) -> (result string=w491:string)  [unwired: 5 in, 3 out]
        n252 = call <vilib>:"Write.vi"("error in (no error)"=w492, "Data"=w491, "WebSocket Connection in"=w493) -> ("error out"=w494:errorcluster, "WebSocket Connection out"=w495:refnum<k5>)  [unwired: 7 in]
        n253 = call <vilib>:"Close.vi"("error in (no error)"=w494, "WebSocket Connection in"=w495) -> ("error out"=w502:errorcluster, "WebSocket Connection in"=w503:refnum<k5>)  [unwired: 8 in]
        n254 = TCP Close Connection(connection ID=w503, error in (no error)=w502) -> (error out=→"error out 3":errorcluster)  [unwired: 1 in, 1 out]
      }
    }
  }
  n255 = while {
    tunnel: w2 -> [w538]
    tunnel: w1 -> [w537]
    stop <- FALSE stop-if-true
    # "Read raptor gps data"
    n256 = Wait Until Next ms Multiple(millisecond multiple=u32 1000 ("milliseconds to wait")) -> ()  [unwired: 1 out]
    n257 = case shown="True" "ROSB READ \ngps raptor" {
      tunnel: w538 -> [_ w544]
      tunnel: w537 -> [_ w543]
      frame False {
      }
      frame True {
        n258 = global read "Gobal for ROS.vi" "String"() -> (w547:string)
        n259 = TCP Open Connection(address="ip raptor", remote port or service name="rosbrige port raptor") -> (connection ID=w563:refnum<k5>, error out=w562:errorcluster)  [unwired: 3 in]
        n260 = TCP Write(connection ID=w563, data in=w547, error in (no error)=w562) -> (connection ID out=w559:refnum<k5>, error out=w558:errorcluster)  [unwired: 1 in, 1 out]
        n261 = call <vilib>:"Write.vi"("error in (no error)"=w558, "Data"="Topic string 4", "WebSocket Connection in"=w559) -> ("error out"=w556:errorcluster, "WebSocket Connection out"=w557:refnum<k5>)  [unwired: 7 in]
        n262 = while {
          tunnel: [w583] -> w553
          tunnel: [w565] -> w552
          tunnel: w557 -> [w584]
          tunnel: w556 -> [w581]
          tunnel: w544 -> [w574]
          tunnel: w543 -> [w573]
          stop <- w575 stop-if-true
          n263 = Get Notifier Status(notifier=w574, error in (no error)=w573) -> (current notification=w572:bool)  [unwired: 4 out]
          n264 = call "ROSBRIDGE TCP READ.vi"("error in (no error)"=w581, "String in"="", "TCP Network Connection in"=w584) -> ("error out"=w582:errorcluster, "String out"=w579:string, "TCP Network Connection out"=w583:refnum<k5>)  [unwired: 6 in]
          "raw frame 6" <- w579
          n265 = Unflatten From JSON(JSON string=w579, type and defaults=T11 {"topic"="", "msg"={"header"={"seq"=0, "stamp"={"secs"=0, "nsecs"=0}, "frame_id"=""}, "status"={"status"=0, "service"=0}, "position_covariance"=[], "latitude"=0.0, "longitude"=0.0, "altitude"=0.0, "position_covariance_type"=0.0}, "op"=""} ("ROS data read 3"), default null elements? (F)=TRUE, error in (no error)=w582) -> (value=w578:T11, error out=w565:errorcluster)  [unwired: 3 in]
          "ROS data read 5" <- w578
          n266 = Unbundle By Name(w578) -> ("msg.latitude"=w570:dbl, "msg.longitude"=w569:dbl, "msg.altitude"=w568:dbl)
          n267 = global read "azymut.vi" "azymut"() -> (w564:dbl)
          n268 = global write "longitude.vi" "Longitude"(w569) -> ()
          n269 = global write "latitude.vi" "latitude"(w570) -> ()
          n270 = Wait Until Next ms Multiple(millisecond multiple=u32 5) -> ()  [unwired: 1 out]
          n271 = call "Wyznaczenie azymutu na podstawie współrzędnych geograficznych.vi"("latitude"=w570, "Longitude"=w569) -> ("Azymut robota\n pocz/nowy 2"=w577:dbl)  [unwired: 9 in]
          n272 = call "Elapsed Time"() -> ("Time has Elapsed"=w567:bool)  [unwired: 12 in, 7 out]
          n273 = Select(t=w577, s=w572, f=w564) -> (s? t:f=w571:dbl)
          n274 = case shown="True" w567 {
            tunnel: w571 -> [_ w592]
            tunnel: w570 -> [_ w591]
            tunnel: w569 -> [_ w590]
            tunnel: w568 -> [_ w589]
            frame False {
            }
            frame True {
              n275 = Number To Fractional String(number=w592) -> (F-format string=w597:string)  [unwired: 3 in]
              n276 = Number To Fractional String(number=w591) -> (F-format string=w596:string)  [unwired: 3 in]
              n277 = Number To Fractional String(number=w590) -> (F-format string=w594:string)  [unwired: 3 in]
              n278 = Number To Fractional String(number=w589) -> (F-format string=w595:string)  [unwired: 3 in]
              n279 = call "UTC KML time.vi"() -> ("String"=w593:string)  [unwired: 19 in]
              n280 = Build Array(w597, w596, w595, w594, T10 "UGV1-Raptor" ("List of robots"), w593) -> (w587:T10[])
              n281 = call "Zapis tabeli do pliku.vi"("1d array in"=w587) -> ("for 1d array out"=w601:string)  [unwired: 7 in, 1 out]
              n282 = Read from Text File(file (use dialog)="UGV1-Raptor") -> (text=w598:string)  [unwired: 3 in, 3 out]
              n283 = Concatenate Strings(w598, w601) -> (w599:string)
              n284 = Write to Text File(file (use dialog)="UGV1-Raptor", text=w599) -> ()  [unwired: 2 in, 3 out]
            }
          }
          n285 = Or(x=w565, y="STOP ROS READ\ngps raptor") -> (x .or. y?=w575:bool)
        }
        n286 = Search and Replace String(input string="Topic string 4", search string="subscribe", replace string="unsubscribe" ("search string")) -> (result string=w551:string)  [unwired: 5 in, 3 out]
        n287 = call <vilib>:"Write.vi"("error in (no error)"=w552, "Data"=w551, "WebSocket Connection in"=w553) -> ("error out"=w554:errorcluster, "WebSocket Connection out"=w555:refnum<k5>)  [unwired: 7 in]
        n288 = call <vilib>:"Close.vi"("error in (no error)"=w554, "WebSocket Connection in"=w555) -> ("error out"=w560:errorcluster, "WebSocket Connection in"=w561:refnum<k5>)  [unwired: 8 in]
        n289 = TCP Close Connection(connection ID=w561, error in (no error)=w560) -> (error out=→"error out 6":errorcluster)  [unwired: 1 in, 1 out]
      }
    }
  }
  n290 = while {
    tunnel: w16 -> [w603]
    tunnel: w15 -> [w602]
    stop <- FALSE stop-if-true
    # "Read UAV-2 gps"
    n291 = Wait Until Next ms Multiple(millisecond multiple=u32 1000 ("milliseconds to wait")) -> ()  [unwired: 1 out]
    n292 = case shown="True" "ROSB READ \ngps dron 2" {
      tunnel: w603 -> [_ w608]
      tunnel: w602 -> [_ w607]
      frame False {
      }
      frame True {
        n293 = global read "Gobal for ROS.vi" "String"() -> (w609:string)
        n294 = TCP Open Connection(address="ip dron 2", remote port or service name="rosbrige port  dron 2") -> (connection ID=w628:refnum<k5>, error out=w627:errorcluster)  [unwired: 3 in]
        n295 = TCP Write(connection ID=w628, data in=w609, error in (no error)=w627) -> (connection ID out=w624:refnum<k5>, error out=w623:errorcluster)  [unwired: 1 in, 1 out]
        n296 = call <vilib>:"Write.vi"("error in (no error)"=w623, "Data"="Topic string 7", "WebSocket Connection in"=w624) -> ("error out"=w621:errorcluster, "WebSocket Connection out"=w622:refnum<k5>)  [unwired: 7 in]
        n297 = while {
          tunnel: [w658] -> w618
          tunnel: [w649] -> w617
          tunnel: w622 -> [w659]
          tunnel: w621 -> [w656]
          tunnel: w608 -> [w646]
          tunnel: w607 -> [w645]
          stop <- w647 stop-if-true
          n298 = call "ROSBRIDGE TCP READ.vi"("error in (no error)"=w656, "String in"="", "TCP Network Connection in"=w659) -> ("error out"=w657:errorcluster, "String out"=w654:string, "TCP Network Connection out"=w658:refnum<k5>)  [unwired: 6 in]
          "raw frame 8" <- w654
          n299 = Unflatten From JSON(JSON string=w654, type and defaults=T6 {"topic"="/drone1/gps", "op"="publish", "msg"={"header"={"seq"=404, "stamp"={"secs"=1505897851, "nsecs"=832105807}, "frame_id"="fcu"}, "status"={"status"=0, "service"=1}, "position_covariance"=[0.0, 0.0, 0.0, 0.0, 0.0, 0.0, 0.0, 0.0, 0.0], "latitude"=47.3977423, "longitude"=8.5455944, "altitude"=0.08040245622396469, "position_covariance_type"=1.0}} ("ROS data read 8"), default null elements? (F)=TRUE, error in (no error)=w657) -> (value=w652:T6, error out=w649:errorcluster)  [unwired: 3 in]
          "ROS data read 7" <- w652
          n300 = Get Notifier Status(notifier=w646, error in (no error)=w645) -> (current notification=w644:bool)  [unwired: 4 out]
          n301 = local read "msg.heading"() -> (w650:dbl)
          n302 = Unbundle By Name(w652) -> ("msg.latitude"=w631:dbl, "msg.longitude"=w630:dbl, "msg.altitude"=w629:dbl)
          n303 = call "Wyznaczenie azymutu na podstawie współrzędnych geograficznych.vi"("latitude"=w631, "Longitude"=w630) -> ("Azymut robota\n pocz/nowy 2"=w651:dbl)  [unwired: 9 in]
          n304 = global write "Longitude dron 2.vi" "Longitude dron 2"(w630) -> ()
          n305 = global write "Latitude dron 2.vi" "Latitude dron 2"(w631) -> ()
          n306 = Select(t=w651, s=w644, f=w650) -> (s? t:f=w632:dbl)
          n307 = Or(x=w649, y="STOP ROS READ \ngps dron 2") -> (x .or. y?=w647:bool)
          n308 = Number To Fractional String(number=w632) -> (F-format string=w639:string)  [unwired: 3 in]
          n309 = Number To Fractional String(number=w631) -> (F-format string=w638:string)  [unwired: 3 in]
          n310 = Number To Fractional String(number=w630) -> (F-format string=w636:string)  [unwired: 3 in]
          n311 = Number To Fractional String(number=w629) -> (F-format string=w637:string)  [unwired: 3 in]
          n312 = call "UTC KML time.vi"() -> ("String"=w635:string)  [unwired: 19 in]
          n313 = Build Array(w639, w638, w637, w636, T10 "UGV1-Raptor" ("List of robots"), w635) -> (w633:T10[])
          n314 = call "Zapis tabeli do pliku.vi"("1d array in"=w633) -> ("for 1d array out"=w640:string)  [unwired: 7 in, 1 out]
          n315 = Read from Text File(file (use dialog)="UAV-2") -> (text=w643:string)  [unwired: 3 in, 3 out]
          n316 = Concatenate Strings(w643, w640) -> (w642:string)
          n317 = Write to Text File(file (use dialog)="UAV-2", text=w642) -> ()  [unwired: 2 in, 3 out]
        }
        n318 = Search and Replace String(input string="Topic string 7", search string="subscribe", replace string="unsubscribe" ("search string")) -> (result string=w616:string)  [unwired: 5 in, 3 out]
        n319 = call <vilib>:"Write.vi"("error in (no error)"=w617, "Data"=w616, "WebSocket Connection in"=w618) -> ("error out"=w619:errorcluster, "WebSocket Connection out"=w620:refnum<k5>)  [unwired: 7 in]
        n320 = call <vilib>:"Close.vi"("error in (no error)"=w619, "WebSocket Connection in"=w620) -> ("error out"=w625:errorcluster, "WebSocket Connection in"=w626:refnum<k5>)  [unwired: 8 in]
        n321 = TCP Close Connection(connection ID=w626, error in (no error)=w625) -> (error out=→"error out 11":errorcluster)  [unwired: 1 in, 1 out]
      }
    }
  }
